vi "R.vi"() -> ()   [LabVIEW 2020]
panel:
  out "R":dbl
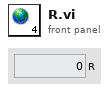
[diagram p1: front panel]
diagram:
